vi "ukol1.vi"() -> ()   [LabVIEW 2023]
uses:
  <vilib>/addons/Digital Filter Design/Process.llb/DFD Filtering with State (Wfm).vi
  <vilib>/Analysis/NI_AALPro.lvlib
  <vilib>/addons/Digital Filter Design/NI_DigFilterLicensed.lvlib
  <vilib>/measure/NI_MABase.lvlib
panel:
  in  "stop":bool
  out "hilbert 4":waveform(dbl)(graph)
  out "hilbert 3":dbl[](graph)
  out "hold 2":dbl[](graph)
  in  "Noise STD":dbl format="%.2p"
  out "hold":waveform(dbl)(graph)
  out "hilbert 2":waveform(dbl)(graph)
  out "vsechny":waveform(dbl)[](graph)
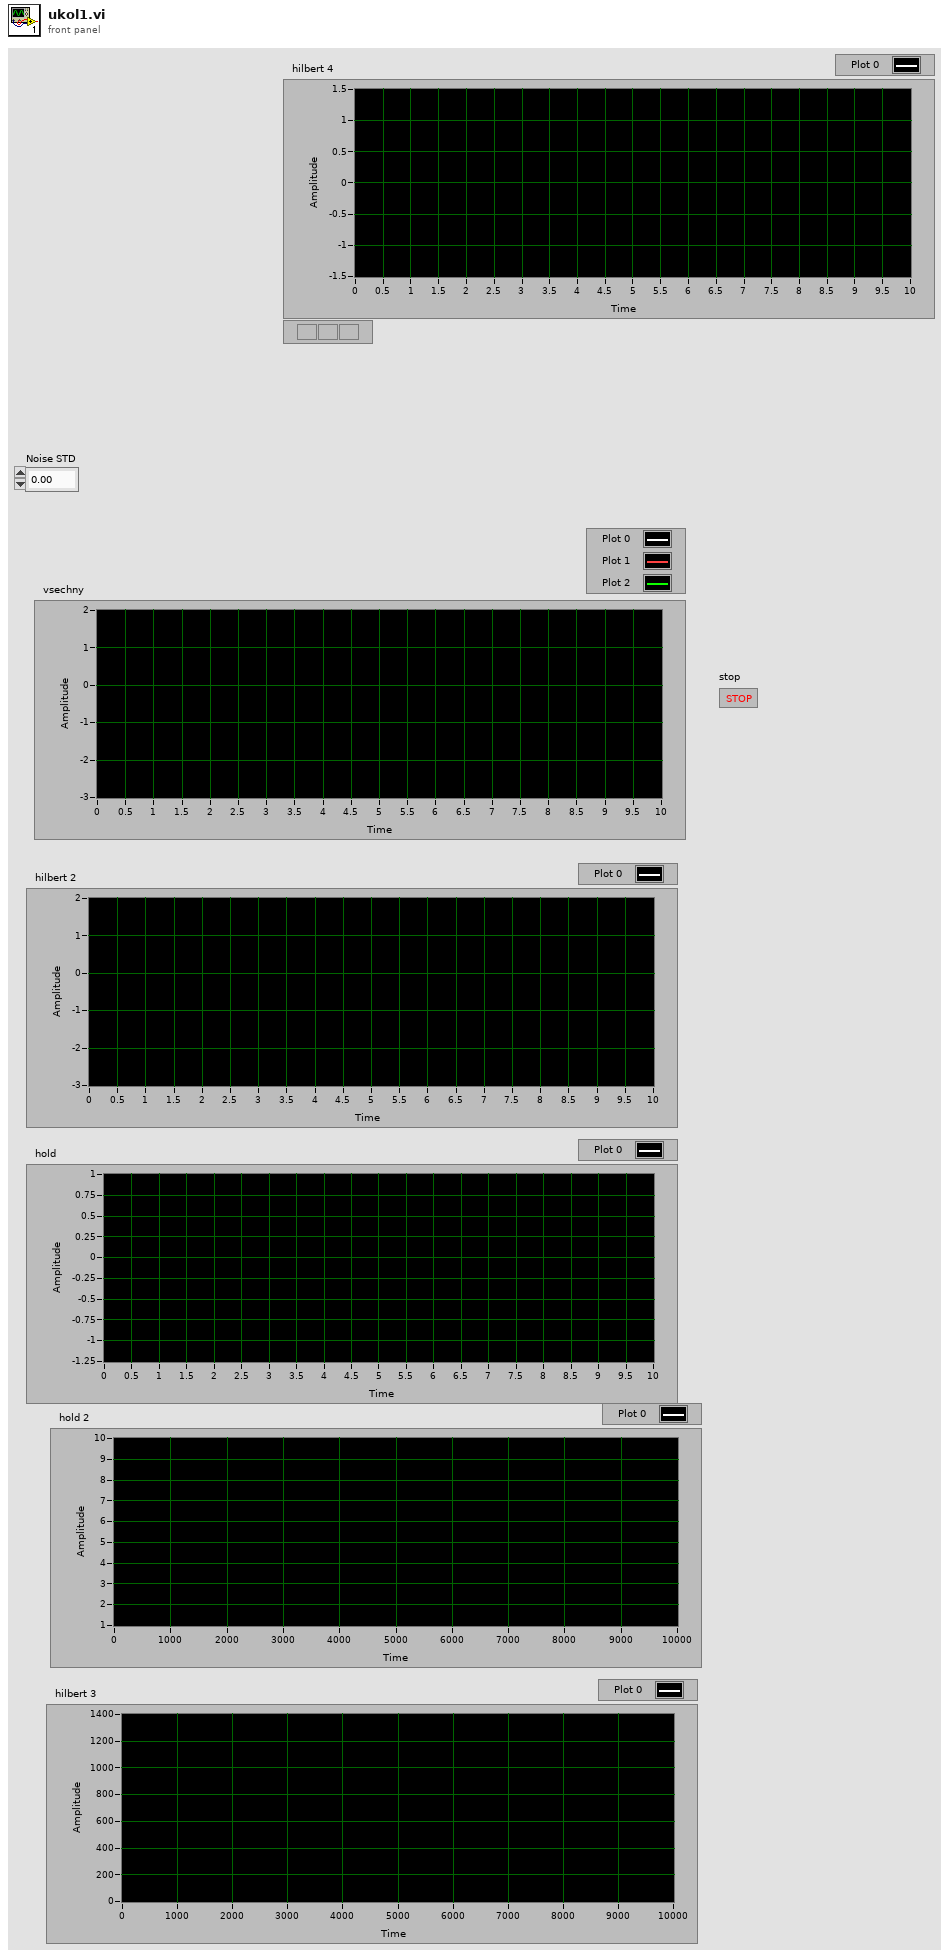
[diagram p1: front panel]
types:
  T1 = typedef "NI_DigFilterLicensed.lvlib/DFD Filter Obj.ctl" = cluster{"mSRate_Fs":dbl, "mSRate_Version":string, "mSRate_Comments":string, "mSRate_OrgCoef":T2, "mSRate_CurCoef":T2, "mSRate_Quantized?":bool, "mSRate_QCoef":T2, "mSRate_QSettings":T4[], "mSRate_Order":i32, "mSRate_Scaling":cluster{"mSRate_ScaleByPowerOf2?":bool, "mSRate_ScaleType":T6}}
  T2 = typedef "NI_DigFilterLicensed.lvlib/DFD Filter Coef.ctl" = cluster{"type":T3, "gain":dbl, "coef a (k)":dbl[], "coef b (v)":dbl[]}
  T3 = typedef "NI_DigFilterLicensed.lvlib/DFD Filter Structure Type Selector.ctl" = enum16{"Undefined", "FIR Direct Form", "FIR Direct Form Transposed", "FIR Symmetric", "FIR Antisymmetric", "IIR Direct Form I", "IIR Direct Form I Transposed", "IIR Direct Form II", "IIR Direct Form II Transposed", "IIR Cascaded Second Order Sections Form I", "IIR Cascaded Second Order Sections Form I Transposed", "IIR Cascaded Second Order Sections Form II", "IIR Cascaded Second Order Sections Form II Transposed", "Lattice Allpass (basic sections)", "Lattice Allpass (one multiplier sections)", "Lattice Allpass (normalized sections)", "Lattice AR (basic sections)", "Lattice AR (one multiplier sections)", "Lattice AR (normalized sections)", "Lattice MA (minimum phase)", "Lattice MA (maximum phase)", "Lattice ARMA (basic sections)", "Lattice ARMA (one multiplier sections)", "Lattice ARMA (normalized sections)"}
  T4 = typedef "NI_DigFilterLicensed.lvlib/dfd_Internal Quantization Settings.ctl" = cluster{"source":T5, "wl":i16, "iwl":i16, "overflow mode":enum16{"Saturation", "Wrap"}, "rounding mode":enum16{"Nearest", "Truncation"}, "signed?":bool}
  T5 = typedef "NI_DigFilterLicensed.lvlib/dfd_Internal Quantization Srcs.ctl" = u16
  T6 = typedef "NI_DigFilterLicensed.lvlib/DFD Coef Norm Type.ctl" = enum16{"No Norm", "Time Domain 1-Norm", "Time Domain 2-Norm", "Time Domain Inf-Norm"}
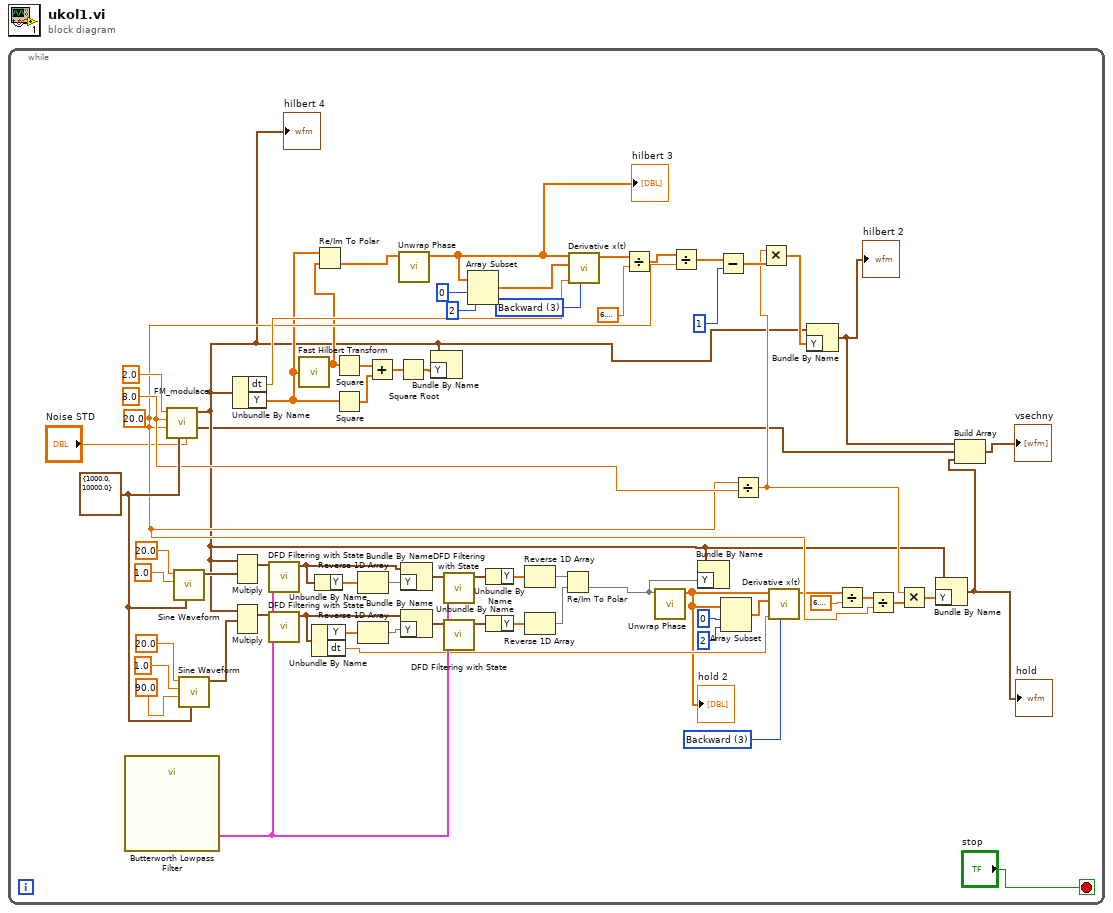
[diagram p0: block diagram]
diagram:
  n1 = while {
    stop <- "stop" stop-if-true
    w32 = u16 3 items=["2nd Order Central", "4th Order Central", "Forward", "Backward"] ("method")
    w40 = u16 3 items=["2nd Order Central", "4th Order Central", "Forward", "Backward"] ("method")
    w46 = cluster{"Fs":dbl, "#s":dbl} {"Fs"=1000.0, "#s"=10000.0} ("Sampling info")
    w28 = 20.0 ("Nosna Frekvence (Hz)")
    w29 = 8.0 ("Frekvencni zdvih (Hz)")
    n2 = call "Butterworth Lowpass Filter"() -> ("filter out"=w41:T1)  [unwired: 10 in, 1 out]
    n3 = call "FM_modulace.vi"("Noise STD"="Noise STD", "Sampling info"=w46, "Nosna Frekvence (Hz)"=w28, "Frekvencni zdvih (Hz)"=w29, "Modulacni Frekvence (Hz)"=2.0) -> ("Modulacni signal"=w3:waveform(dbl), "Modulovany signal"=w5:waveform(dbl))  [unwired: 3 in, 2 out]
    "hilbert 4" <- w5
    n4 = call <vilib>:"Sine Waveform.vi"("sampling info"=w46, "amplitude"=1.0, "frequency"=20.0) -> ("signal out"=w45:waveform(dbl))  [unwired: 7 in, 1 out]
    n5 = call <vilib>:"Sine Waveform.vi"("sampling info"=w46, "phase"=90.0, "amplitude"=1.0, "frequency"=20.0) -> ("signal out"=w44:waveform(dbl))  [unwired: 6 in, 1 out]
    n6 = Multiply(1:w45, 2:w5) -> (0:w43:waveform(dbl))  [unwired: 1 in, 1 out]
    n7 = Multiply(1:w44, 2:w5) -> (0:w42:waveform(dbl))  [unwired: 1 in, 1 out]
    n8 = Unbundle By Name(w5) -> ("dt"=w39:dbl, "Y"=w8:dbl[])
    n9 = call-poly <vilib>:"DFD Filtering with State.vi"("filter"=w41, "signal in"=w43) -> ("signal out"=w55:waveform(dbl))  [unwired: 7 in, 2 out]
    n10 = call-poly <vilib>:"DFD Filtering with State.vi"("filter"=w41, "signal in"=w42) -> ("signal out"=w61:waveform(dbl))  [unwired: 7 in, 2 out]
    n11 = call <vilib>:"Fast Hilbert Transform.vi"("X"=w8) -> ("Hilbert{X}"=w7:dbl[])  [unwired: 1 out]
    n12 = Unbundle By Name(w61) -> ("Y"=w63:dbl[], "dt"=w18:dbl)
    n13 = Re/Im To Polar(2:w7, 3:w8) -> (0:w6:dbl[])  [unwired: 1 out]
    n14 = Unbundle By Name(w55) -> ("Y"=w57:dbl[])
    n15 = Square(x=w7) -> (x^2=w67:dbl[])
    n16 = Square(x=w8) -> (x^2=w66:dbl[])
    n17 = Reverse 1D Array(array=w57) -> (reversed array=w56:dbl[])
    n18 = Reverse 1D Array(array=w63) -> (reversed array=w62:dbl[])
    n19 = Add(x=w67, y=w66) -> (x+y=w65:dbl[])
    n20 = Square Root(x=w65) -> (sqrt(x)=w64:dbl[])
    n21 = call <vilib>:"Unwrap Phase.vi"("Phase"=w6) -> ("Unwrapped Phase"=w9:dbl[])  [unwired: 9 in, 1 out]
    "hilbert 3" <- w9
    n22 = Bundle By Name(cluster=w55, "Y"=w56) -> (w54:waveform(dbl))
    n23 = Bundle By Name(cluster=w61, "Y"=w62) -> (w60:waveform(dbl))
    n24 = Bundle By Name(cluster=w5, "Y"=w64) -> ()  [unwired: 1 out]
    n25 = call-poly <vilib>:"DFD Filtering with State.vi"("filter"=w41, "signal in"=w54) -> ("signal out"=w52:waveform(dbl))  [unwired: 7 in, 2 out]
    n26 = call-poly <vilib>:"DFD Filtering with State.vi"("filter"=w41, "signal in"=w60) -> ("signal out"=w58:waveform(dbl))  [unwired: 7 in, 2 out]
    n27 = Array Subset(array=w9, index=0, length=2) -> (w11:dbl[])
    n28 = Unbundle By Name(w52) -> ("Y"=w53:dbl[])
    n29 = Unbundle By Name(w58) -> ("Y"=w59:dbl[])
    n30 = Reverse 1D Array(array=w53) -> (reversed array=w20:dbl[])
    n31 = Reverse 1D Array(array=w59) -> (reversed array=w19:dbl[])
    n32 = Re/Im To Polar(2:w19, 3:w20) -> (0:w4:dbl[])  [unwired: 1 out]
    n33 = call <vilib>:"Derivative x(t).vi"("method"=w40, "dt"=w39, "Initial Condition"=w11, "X"=w9) -> ("dX/dt"=w22:dbl[])  [unwired: 6 in, 1 out]
    n34 = Divide(x=w22, y=6.283185307179586) -> (x/y=w21:dbl[])
    n35 = call <vilib>:"Unwrap Phase.vi"("Phase"=w4) -> ("Unwrapped Phase"=w10:dbl[])  [unwired: 9 in, 1 out]
    "hold 2" <- w10
    n36 = Divide(x=w21, y=w28) -> (x/y=w38:dbl[])
    n37 = Bundle By Name(cluster=w5, "Y"=w4) -> ()  [unwired: 1 out]
    n38 = Subtract(x=w38, y=1) -> (x-y=w36:dbl[])
    n39 = Array Subset(array=w10, index=0, length=2) -> (w14:dbl[])
    n40 = Divide(x=w28, y=w29) -> (x/y=w27:dbl)
    n41 = Multiply(x=w27, y=w36) -> (x*y=w35:dbl[])
    n42 = call <vilib>:"Derivative x(t).vi"("method"=w32, "dt"=w18, "Initial Condition"=w14, "X"=w10) -> ("dX/dt"=w25:dbl[])  [unwired: 6 in, 1 out]
    n43 = Bundle By Name(cluster=w5, "Y"=w35) -> (w34:waveform(dbl))
    "hilbert 2" <- w34
    n44 = Divide(x=w25, y=6.283185307179586) -> (x/y=w24:dbl[])
    n45 = Divide(x=w24, y=w28) -> (x/y=w30:dbl[])
    n46 = Multiply(x=w27, y=w30) -> (x*y=w31:dbl[])
    n47 = Bundle By Name(cluster=w5, "Y"=w31) -> (w17:waveform(dbl))
    "hold" <- w17
    n48 = Build Array(w34, w3, w17) -> (→"vsechny":waveform(dbl)[])
  }
